vi "Quick_analogInp_View.vi"() -> ()   [LabVIEW 2013]
doc: "I. Description:\nThis example demonstrates how to acquire a continuous amount of data (Waveform) using the DAQ device's internal clock.\n\nII. Instructions for Running:\n1. Create an analog input voltage channel.\n2. Set the rate for the sample clock. Additionally, define the sample mode to be continuous.\n3. Call the Start VI to start the acquisition.\n4. Read the waveform data in a loop until the user hits the stop button or an error occurs.\nNote: This example reads data from one or more channels and returns an array of data. Use the Index Array function to access an individual channel of data.\n5. Call the Clear Task VI to clear the Task.\n6. Use the popup dialog box to display an error if any.\n\nIV. I/O Connections Overview:\nMake sure your signal input terminal matches the Physical Channel I/O Control. For further connection information, refer to your hardware reference manual."
uses:
  <vilib>/Utility/error.llb/DialogType.ctl
  <vilib>/DAQmx/read.llb/DAQmx Read (Analog 2D DBL NChan NSamp).vi
  <vilib>/DAQmx/create/channels.llb/DAQmx Create Channel (AI-Voltage-Basic).vi
  <vilib>/DAQmx/configure/timing.llb/DAQmx Timing (Sample Clock).vi
  <vilib>/DAQmx/miscellaneous.llb/DAQmx Fill In Error Info.vi
panel:
  out "Array of Data":dbl[][](array[numeric])
  in  "Latch Data":bool
  in  "Samples to Read":i32=100
  in  "Physical Channels":tag="PCI-6251/ai2:1" caption="Physical Channel"
  in  "Minimum Value":dbl format="%0.2f"
  in  "Maximum Value":dbl=0.04 format="%0.2f"
  in  "Sample Rate":dbl=1000.0 caption="Sample Rate (Hz)" format="%0.2f"
  in  "stop":bool
  out "Measurement":dbl[][](graph)
  # "When you press the \"Latch Data\" button, X (Samples to Read) number of data points will be read from each physical channel you have selected and stored in the Array of Data array. \n\nPush Stop to exit the code."
  # "Mechanical Action = Latch when Released"
  # "Channel Parameters"
  # "Timing Parameters"
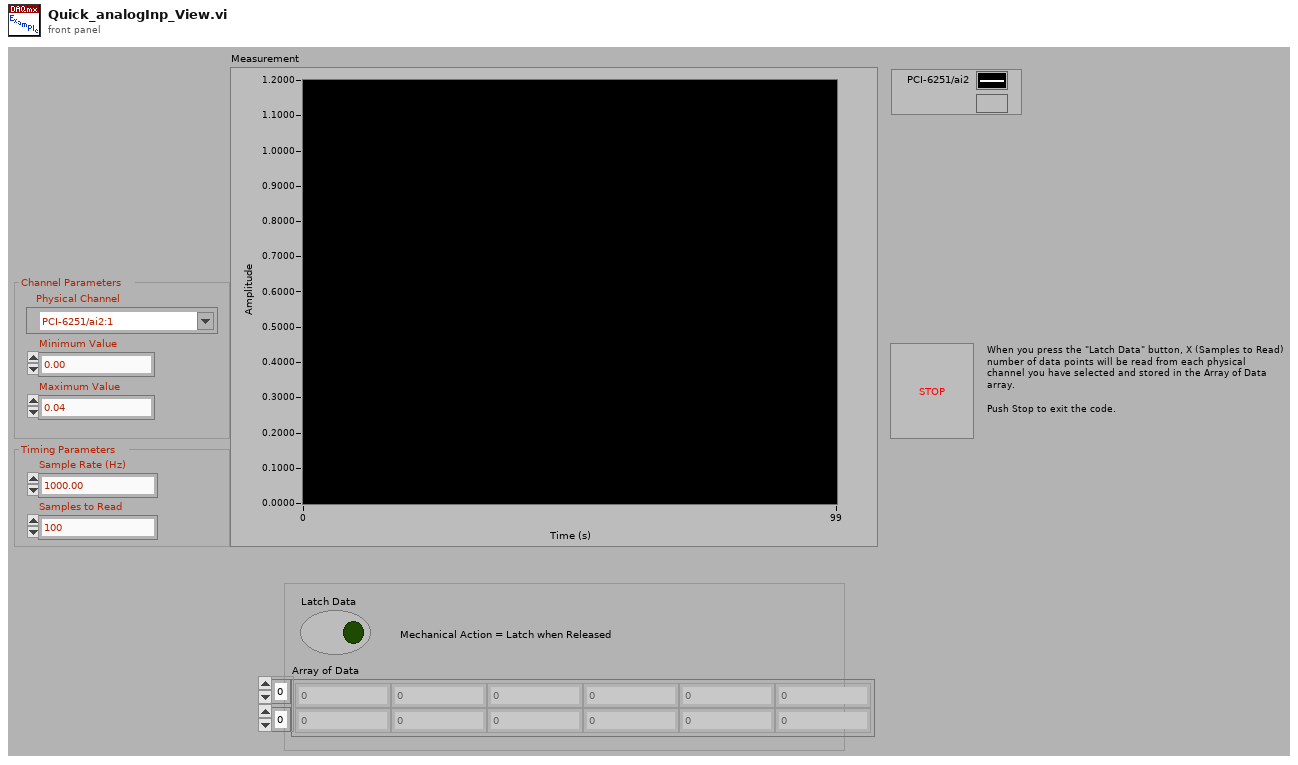
[diagram p1: front panel]
types:
  T1 = typedef "DialogType.ctl" = u16
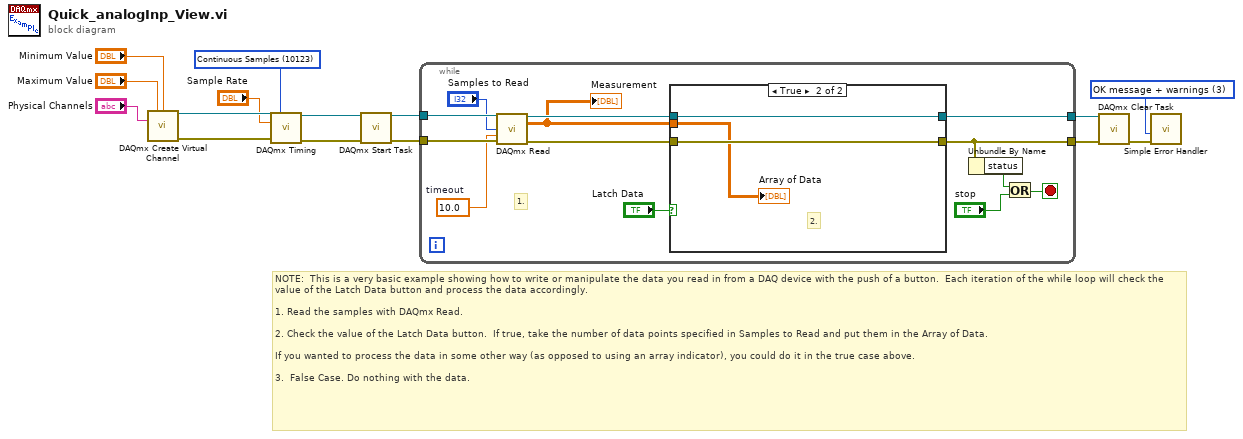
[diagram p0: block diagram]
diagram:
  w1 = T1 3 items=["no dialog", "OK message", "continue or stop message", "OK message + warnings", "continue/stop + warnings"] ("type of dialog (OK msg:1)")
  w6 = 10123 items=["Finite Samples"=10178, "Continuous Samples"=10123] ("sample mode")
  # "NOTE:  This is a very basic example showing how to write or manipulate the data you read in from a DAQ device with the push of a button.  Each iteration of the while loop will check the value of the Latch Data button and process the data accordingly.\n\n1. Read the samples with DAQmx Read.\n\n2. Check the value of the Latch Data button.  If true, take the number of data points specified in Samples to Read and put them in the Array of Data.  \n\nIf you wanted to process the data in some other way (as opposed to using an array indicator), you could do it in the true case above. \n\n3.  False Case. Do nothing with the data."
  n1 = call-poly <vilib>:"DAQmx Create Virtual Channel.vi"("maximum value"="Maximum Value", "minimum value"="Minimum Value", "physical channels"="Physical Channels") -> ("task out"=w10:refnum<k21>, "error out"=w13:errorcluster)  [unwired: 11 in]
  n2 = call-poly <vilib>:"DAQmx Timing.vi"("task/channels in"=w10, "sample mode"=w6, "rate"="Sample Rate", "error in"=w13) -> ("task out"=w5:refnum<k21>, "error out"=w4:errorcluster)  [unwired: 10 in]
  n3 = call <vilib>:"DAQmx Start Task.vi"("task/channels in"=w5, "error in"=w4) -> ("task out"=w9:refnum<k21>, "error out"=w12:errorcluster)  [unwired: 12 in]
  n4 = while {
    tunnel: w12 -> [w28]
    tunnel: w9 -> [w27]
    tunnel: [w20] -> w8
    tunnel: [w18] -> w3
    stop <- w25 stop-if-true
    w23 = 10.0  # timeout
    # "1."
    n5 = call-poly <vilib>:"DAQmx Read.vi"("task/channels in"=w27, "number of samples per channel"="Samples to Read", "timeout"=w23, "error in"=w28) -> ("task out"=w21:refnum<k21>, "data"=w17:dbl[][], "error out"=w19:errorcluster)  [unwired: 9 in]
    "Measurement" <- w17
    n6 = case shown="True" "Latch Data" {
      tunnel: w21 -> [w30 w33]
      tunnel: [w30 w33] -> w20
      tunnel: w19 -> [w29 w32]
      tunnel: [w29 w32] -> w18
      tunnel: w17 -> [_ w31]
      frame False {
        # "3."
      }
      frame True {
        # "2."
        "Array of Data" <- w31
      }
    }
    n7 = Unbundle By Name(w18) -> ("status"=w26:bool)
    n8 = Or(x=w26, y="stop") -> (x .or. y?=w25:bool)
  }
  n9 = call <vilib>:"DAQmx Clear Task.vi"("task in"=w8, "error in"=w3) -> ("error out"=w11:errorcluster)  [unwired: 13 in]
  n10 = call <vilib>:"Simple Error Handler.vi"("type of dialog (OK msg:1)"=w1, "error in (no error)"=w11) -> ()  [unwired: 3 in, 5 out]
